vi "data根路径.vi"() -> (0 "data文件夹":path)   [LabVIEW 2017]
doc: "data数据文件夹, 不存在会自动创建"
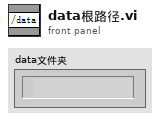
[diagram p1: front panel]
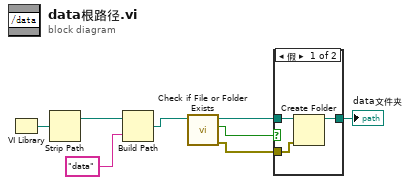
[diagram p0: block diagram]
diagram:
  n1 = VI Library() -> (path=w8:path)
  n2 = Strip Path(path=w8) -> (stripped path=w6:path)  [unwired: 1 out]
  n3 = Build Path(base path=w6, name or relative path="data" ("读报警文件")) -> (appended path=w2:path)
  n4 = call <vilib>:"Check if File or Folder Exists.vi"("path"=w2) -> ("error out"=w3:errorcluster, "file or folder exists?"=w4:bool, "dup path"=w5:path)  [unwired: 8 in]
  n5 = case shown="假" w4 {
    tunnel: w5 -> [w11 w12]
    tunnel: w3 -> [w10 _]
    tunnel: [w9 w12] -> w1
    frame False {
      n6 = Create Folder(path (use dialog)=w11, error in=w10) -> (created path=w9:path)  [unwired: 1 in, 2 out]
    }
    frame True {
    }
  }
  "data文件夹" <- w1
